vi "Module Launch.vi"(6 "VI Path":path, 7 "Parent ID":i32, 8 "error in (no error)":errorcluster, 9 "Config Section":string, 10 "Config Path":path, 11 "Name":string) -> (0 "error out":errorcluster, 2 "VI Refnum":refnum<vi>, 3 "Module":T1)   [LabVIEW 2018, in "Core.lvlib"]
uses:
  Core.lvlib
  Controls/Module Instance.ctl
  Controls/Module.ctl
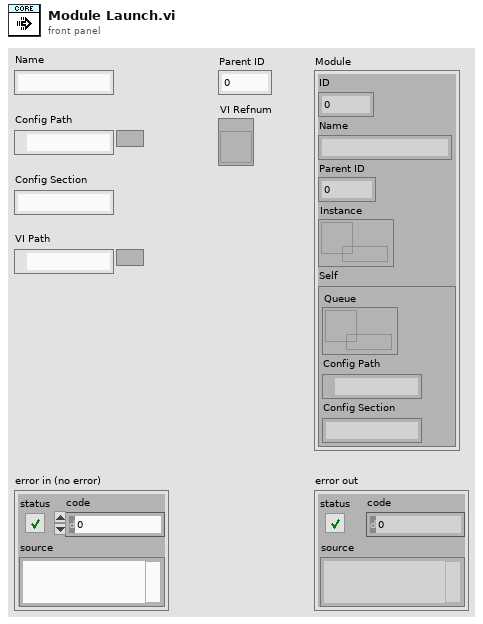
[diagram p1: front panel]
types:
  T1 = typedef "Core.lvlib/Module.ctl" = cluster{"ID":i32, "Name":string, "Parent ID":i32, "Instance":refnum<data-value>, "Self":T2}
  T2 = typedef "Core.lvlib/Module Instance.ctl" = cluster{"Queue":refnum<queue>, "Config Path":path, "Config Section":string}
  T3 = enum32{"Invalid", "Standard", "Closed", "Hidden", "Minimized", "Maximized"}
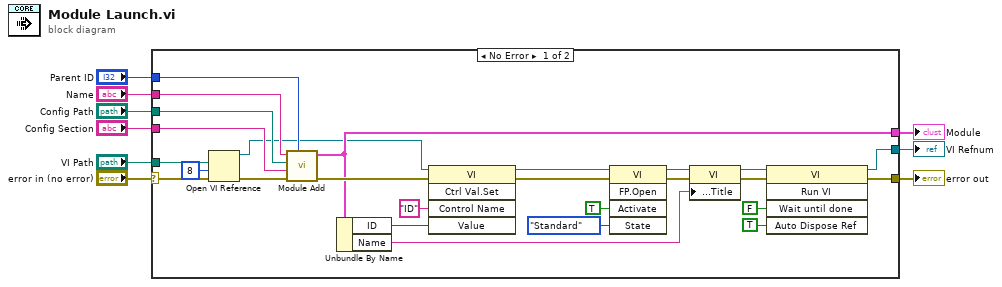
[diagram p0: block diagram]
diagram:
  n1 = case shown="No Error" "error in (no error)" {
    selector: "error in (no error)" -> [w35 w36]
    tunnel: "Parent ID" -> [w34 _]
    tunnel: "Name" -> [w33 _]
    tunnel: "Config Path" -> [w32 _]
    tunnel: "Config Section" -> [w31 _]
    tunnel: [w29 _] -> w4
    tunnel: "VI Path" -> [w27 _]
    tunnel: [w17 w36] -> w2
    tunnel: [w14 _] -> w1
    frame No Error {
      n2 = Open VI Reference(vi path=w27, options=8, error in (no error)=w35) -> (vi reference=w24:refnum<vi>, error out=w28:errorcluster)  [unwired: 3 in]
      n3 = call "Module Add.vi"("Parent ID"=w34, "error in (no error)"=w28, "Config Section"=w31, "Config Path"=w32, "Name"=w33) -> ("error out"=w30:errorcluster, "Module"=w29:T1)  [unwired: 5 in]
      n4 = Unbundle By Name(w29) -> ("ID"=w22:i32, "Name"=w10:string)
      n5 = invoke class="VI" method="Ctrl Val.Set"(reference=w24, error in=w30, "Control Name"="ID", "Value"=w22) -> (reference out=w20:refnum<vi>, error out=w25:errorcluster)  [unwired: 1 in, 3 out]
      n6 = invoke class="VI" method="FP.Open"(reference=w20, error in=w25, "Activate"=TRUE ("Activate?"), "State"=T3."Standard") -> (reference out=w12:refnum<vi>, error out=w21:errorcluster)  [unwired: 1 in, 3 out]
      n7 = property class="VI"(reference=w12, error in=w21, "Front Panel.Title"=w10) -> (reference out=w11:refnum<vi>, error out=w13:errorcluster)
      n8 = invoke class="VI" method="Run VI"(reference=w11, error in=w13, "Wait until done"=FALSE ("Wait Until Done"), "Auto Dispose Ref"=TRUE ("Auto Dispose Reference")) -> (reference out=w14:refnum<vi>, error out=w17:errorcluster)  [unwired: 1 in, 3 out]
    }
    frame Error {
    }
  }
  "error out" <- w2
  "Module" <- w4
  "VI Refnum" <- w1
